vi "E11_M_Garcia_Denise.vi"(10 "Transducer Offset [V]":dbl, 11 "Voltage Input [m/s]":dbl[](array[numeric])) -> (3 "Velocity Output [m/s]":dbl[](array[numeric]))   [LabVIEW 2017]
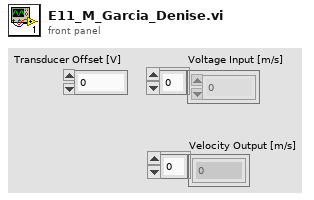
[diagram p1: front panel]
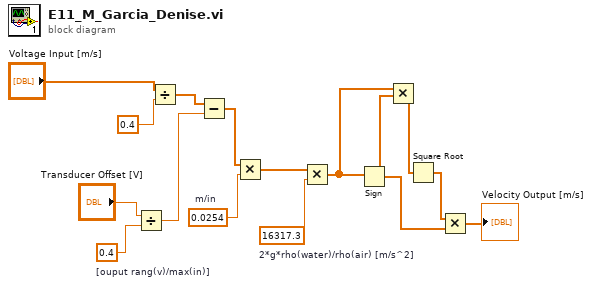
[diagram p0: block diagram]
diagram:
  w7 = 16317.3  # 2*g*rho(water)/rho(air) [m/s^2]
  w8 = 0.0254  # m/in
  w12 = 0.4  # [ouput rang(v)/max(in)]
  n1 = Divide(x="Transducer Offset [V]", y=w12) -> (x/y=w11:dbl)
  n2 = Divide(x="Voltage Input [m/s]", y=0.4) -> (x/y=w14:dbl[])
  n3 = Subtract(x=w14, y=w11) -> (x-y=w10:dbl[])
  n4 = Multiply(x=w10, y=w8) -> (x*y=w6:dbl[])
  n5 = Multiply(x=w6, y=w7) -> (x*y=w5:dbl[])
  n6 = Sign(1:w5) -> (0:w2:dbl[])
  n7 = Multiply(x=w5, y=w2) -> (x*y=w4:dbl[])
  n8 = Square Root(x=w4) -> (sqrt(x)=w3:dbl[])
  n9 = Multiply(x=w3, y=w2) -> (x*y=→"Velocity Output [m/s]":dbl[])
